vi "Flatten Payload.vi"(8 "error in (no error)":errorcluster, 10 "Variant":variant, 11 "IMessagePayload in":refnum<class "IMessagePayload.lvclass">) -> (0 "error out":errorcluster, 3 "IMessagePayload out":refnum<class "IMessagePayload.lvclass">)   [LabVIEW 2016, in "IMessagePayload.lvclass"]
uses:
  IMessagePayload.lvclass
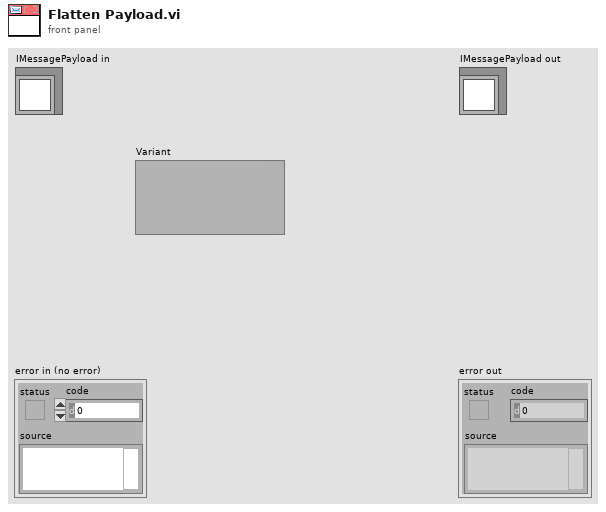
[diagram p1: front panel]
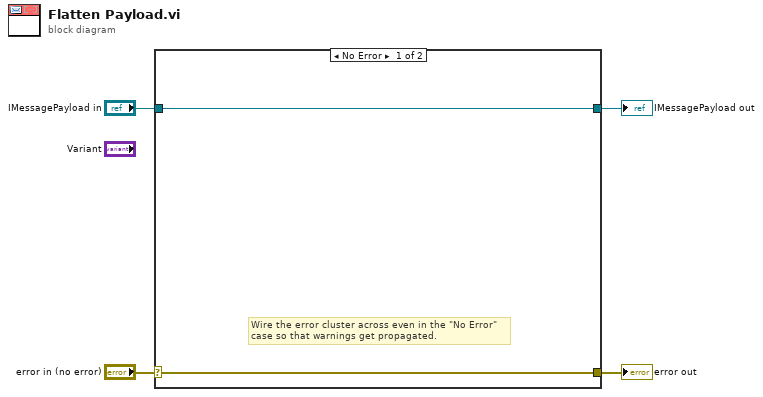
[diagram p0: block diagram]
diagram:
  n1 = case shown="No Error" "error in (no error)" {
    selector: "error in (no error)" -> [w5 w8]
    tunnel: [w5 w8] -> w3
    tunnel: [w6 w7] -> w1
    tunnel: "IMessagePayload in" -> [w6 w7]
    frame No Error {
      # "Wire the error cluster across even in the \"No Error\"\ncase so that warnings get propagated."
    }
    frame Error {
    }
  }
  "error out" <- w3
  "IMessagePayload out" <- w1
